vi "close.vi"(8 "error in (no error)":errorcluster, 11 "WinX32Camera in":refnum<class "WinX32Camera.lvclass">) -> (0 "error out":errorcluster, 3 "WinX32Camera out":refnum<class "WinX32Camera.lvclass">)   [LabVIEW 2011, in "WinX32Camera.lvclass"]
uses:
  WinX32Camera.lvclass
  WinX32Camera.lvclass/WinX32Camera.ctl
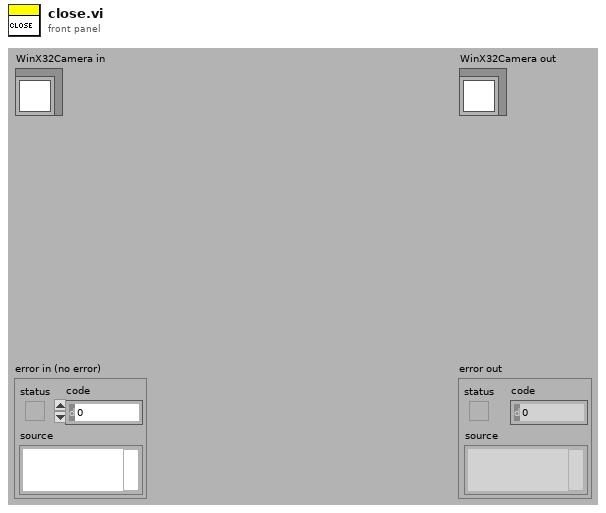
[diagram p1: front panel]
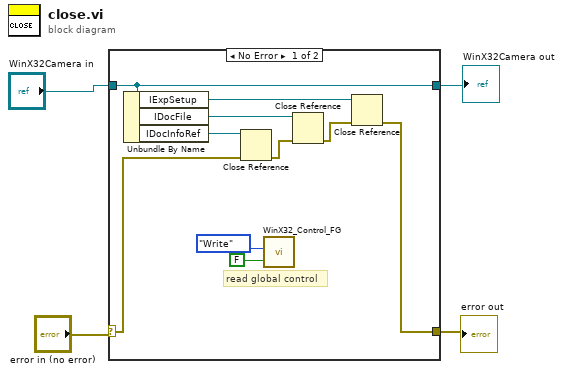
[diagram p0: block diagram]
diagram:
  n1 = case shown="No Error" "error in (no error)" {
    selector: "error in (no error)" -> [w13 w16]
    tunnel: "WinX32Camera in" -> [w12 w15]
    tunnel: [w7 w16] -> w3
    tunnel: [w12 w15] -> w1
    frame No Error {
      # "read global control"
      n2 = Unbundle By Name(w12) -> ("IExpSetup"=w9:refnum<k7>, "IDocFile"=w11:refnum<k7>, "IDocInfoRef"=w14:refnum<k7>)
      n3 = Close Reference(reference=w14, error in (no error)=w13) -> (error out=w10:errorcluster)
      n4 = call "WinX32_Control_FG.vi"("stop"=FALSE, "Action"=enum16{"Write", "Read"}."Write") -> ()  [unwired: 9 in, 1 out]
      n5 = Close Reference(reference=w11, error in (no error)=w10) -> (error out=w8:errorcluster)
      n6 = Close Reference(reference=w9, error in (no error)=w8) -> (error out=w7:errorcluster)
    }
    frame Error {
    }
  }
  "error out" <- w3
  "WinX32Camera out" <- w1
